vi "Obtain SPI.vi"(6 "SPI Config":T1={"Mode"=0, "Data Bits"=8, "TX GPIO"=7, "RX GPIO"=4, "SCK GPIO"=6}, 7 "SPI #":T4=-1, 8 "error in (no error)":errorcluster, 10 "Baud":u32=1000000 format="%.0p", 11 "Session in":refnum<class "Session.lvclass">) -> (0 "error out":errorcluster, 2 "SPI":refnum<class "SPI.lvclass">, 3 "Session out":refnum<class "Session.lvclass">)   [LabVIEW 2020, in "CTI.lvlib" / "Session.lvclass"]
uses:
  Session.lvclass
  Session.lvclass/Session.ctl
  SPI Number.ctl
  CTI.lvlib
  GPIO Number.ctl
  SPI Mode.ctl
  SPI Config.ctl
  SPI/SPI.lvclass
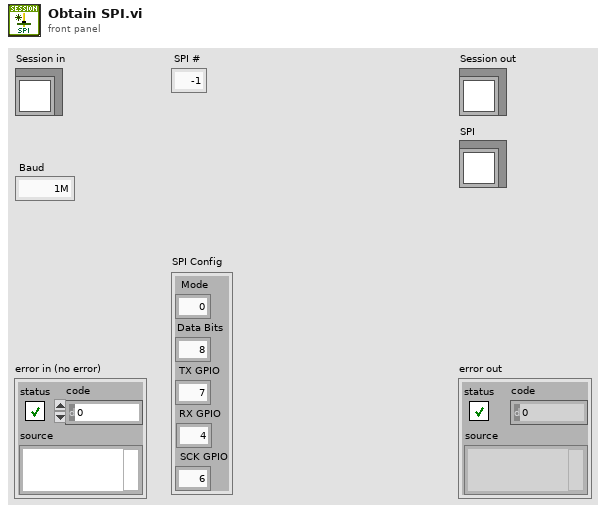
[diagram p1: front panel]
types:
  T1 = typedef "CTI.lvlib/SPI Config.ctl" = cluster{"Mode":T2, "Data Bits":i8, "TX GPIO":T3, "RX GPIO":T3, "SCK GPIO":T3}
  T2 = typedef "CTI.lvlib/SPI Mode.ctl" = i8
  T3 = typedef "CTI.lvlib/GPIO Number.ctl" = i8
  T4 = typedef "CTI.lvlib/SPI Number.ctl" = i8
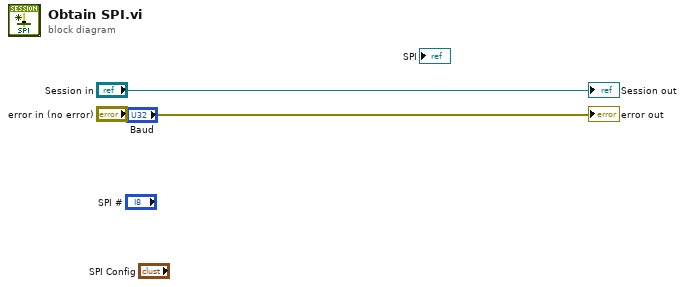
[diagram p0: block diagram]
diagram:
  "error out" <- "error in (no error)"
  "Session out" <- "Session in"
